vi "_script_set_csm_doc_case_as_default.vi"(11 "Vi Path":path=path "D:/github/JKI-State-Machine-Plus/src/user.lib/_NEVSTOP/JKI State Machine++/JKISM++ No-Event Structure Template.vi") -> (0 "error out":errorcluster)   [LabVIEW 2017]
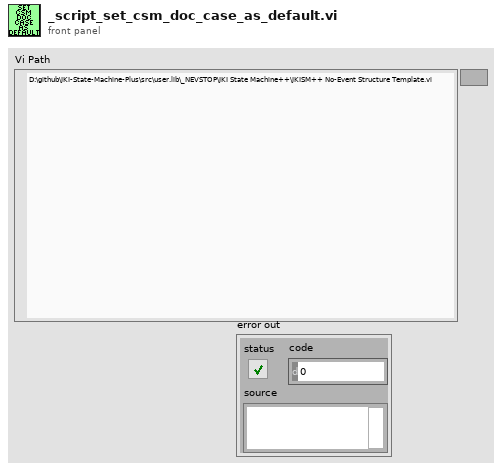
[diagram p1: front panel]
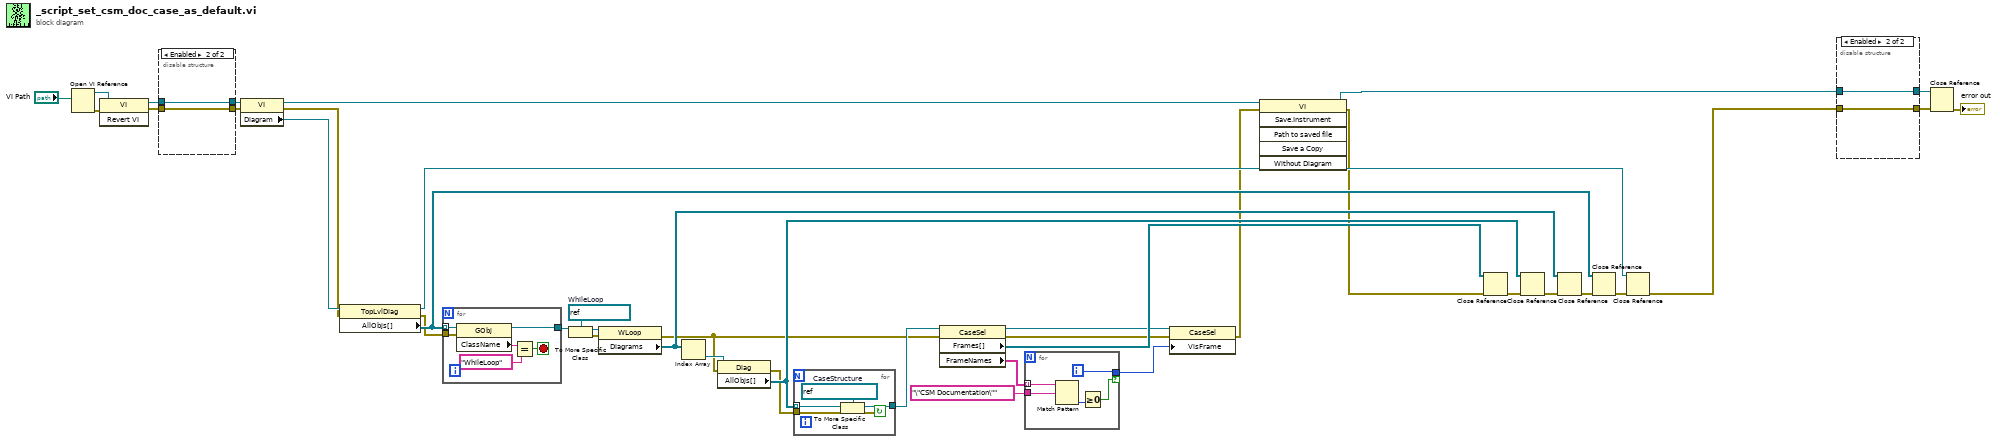
[diagram p0: block diagram]
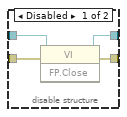
[diagram p2: hidden frame]
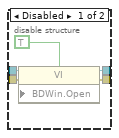
[diagram p3: hidden frame]
diagram:
  w14 = refnum<vi> refnum  # WhileLoop
  n1 = Open VI Reference(vi path="Vi Path") -> (vi reference=w39:refnum<vi>, error out=w40:errorcluster)  [unwired: 5 in]
  n2 = invoke class="VI" method="Revert VI"(reference=w39, error in=w40) -> (reference out=w32:refnum<vi>, error out=w31:errorcluster)  [unwired: 1 in, 1 out]
  n3 = disable-structure shown="Enabled" {
    disable-tunnel: w32 -> [w45 w47]
    disable-tunnel: w31 -> [w44 w46]
    disable-tunnel: [w43 w47] -> w30
    disable-tunnel: [w42 w46] -> w29
    frame Disabled {
      n4 = property class="VI"(reference=w45, error in=w44, "BDWin.Open"=TRUE ("Block Diagram Window:Open")) -> (reference out=w43:refnum<vi>, error out=w42:errorcluster)
    }
    frame Enabled {
    }
  }
  n5 = property class="VI"(reference=w30, error in=w29) -> (reference out=w19:refnum<vi>, error out=w37:errorcluster, "Diagram"=w38:refnum<vi>)
  n6 = property class="TopLvlDiag"(reference=w38, error in=w37) -> (reference out=w33:refnum<vi>, error out=w16:errorcluster, "AllObjs[]"=w35:refnum<vi>[])
  n7 = for {
    tunnel: w35 -> [w53] mode=indexing
    tunnel: w16 -> [w52]
    tunnel: [w51] -> w15
    stop <- w48 stop-if-true
    n8 = property class="GObj"(reference=w53, error in=w52) -> (reference out=w51:refnum<vi>, "ClassName"=w50:string)  [unwired: 1 out]
    n9 = Equal?(x=w50, y="WhileLoop") -> (x = y?=w48:bool)
  }
  n10 = To More Specific Class(target class=w14, reference=w15) -> (specific class reference=w13:refnum<vi>, error out=w12:errorcluster)  [unwired: 1 in]
  n11 = property class="WLoop"(reference=w13, error in=w12) -> (error out=w8:errorcluster, "Diagrams"=w28:refnum<vi>[])  [unwired: 1 out]
  n12 = Index Array(array=w28) -> (element=w11:refnum<vi>)  [unwired: 1 in]
  n13 = property class="Diag"(reference=w11, error in=w8) -> (error out=w10:errorcluster, "AllObjs[]"=w25:refnum<vi>[])  [unwired: 1 out]
  n14 = for {
    tunnel: w25 -> [w58] mode=indexing
    tunnel: w10 -> [w57]
    tunnel: [w55] -> w9
    stop <- w56 continue-if-true
    w54 = refnum<vi> refnum  # CaseStructure
    n15 = To More Specific Class(target class=w54, reference=w58, error in=w57) -> (specific class reference=w55:refnum<vi>, error out=w56:errorcluster)
  }
  n16 = property class="CaseSel"(reference=w9, error in=w8) -> (reference out=w5:refnum<vi>, error out=w4:errorcluster, "Frames[]"=w23:refnum<vi>[], "FrameNames"=w7:string[])
  n17 = for {
    tunnel: w7 -> [w63] mode=indexing
    tunnel: [w62] -> w2 if=w60
    tunnel: "\"CSM Documentation\"" ("regular expression") -> [w59]
    i -> [w62]
    n18 = Match Pattern(string=w63, regular expression=w59) -> (offset past match=w61:i32)  [unwired: 1 in, 3 out]
    n19 = Greater Or Equal To 0?(x=w61) -> (x >= 0?=w60:bool)
  }
  n20 = property class="CaseSel"(reference=w5, error in=w4, "VisFrame"=w2) -> (error out=w3:errorcluster)  [unwired: 1 out]
  n21 = invoke class="VI" method="Save.Instrument"(reference=w19, error in=w3) -> (reference out=w21:refnum<vi>, error out=w18:errorcluster)  [unwired: 4 in, 4 out]
  n22 = Close Reference(reference=w23, error in (no error)=w18) -> (error out=w27:errorcluster)
  n23 = Close Reference(reference=w25, error in (no error)=w27) -> (error out=w26:errorcluster)
  n24 = Close Reference(reference=w28, error in (no error)=w26) -> (error out=w36:errorcluster)
  n25 = Close Reference(reference=w35, error in (no error)=w36) -> (error out=w34:errorcluster)
  n26 = Close Reference(reference=w33, error in (no error)=w34) -> (error out=w17:errorcluster)
  n27 = disable-structure shown="Enabled" {
    disable-tunnel: [w67 w69] -> w22
    disable-tunnel: w21 -> [w66 w68]
    disable-tunnel: [w65 w68] -> w20
    disable-tunnel: w17 -> [w64 w69]
    frame Disabled {
      n28 = invoke class="VI" method="FP.Close"(reference=w66, error in=w64) -> (reference out=w65:refnum<vi>, error out=w67:errorcluster)  [unwired: 1 in, 1 out]
    }
    frame Enabled {
    }
  }
  n29 = Close Reference(reference=w20, error in (no error)=w22) -> (error out=→"error out":errorcluster)
